vi "alphanumkey_pw.vi"(8 "error in (no error)":errorcluster, 11 "Old Input":string) -> (0 "error out":errorcluster, 3 "Output String":string)   [LabVIEW 2014]
doc: "This VI serves as an on screen keyboard for touch panel modules."
panel:
  in  "Cancel Button":bool
  in  "OK Button":bool
  in  "Boolean":bool
  in  "*":bool
  in  "Delete":bool
  in  "#":bool
  in  "0":bool
  in  ".":bool
  in  "9":bool
  in  "8":bool
  in  "7":bool
  in  "6":bool
  in  "5":bool
  in  "4":bool
  in  "3":bool
  in  "2":bool
  in  "1":bool
  in  "RShift":bool
  in  "Z":bool
  in  "Y":bool
  in  "X":bool
  in  "W":bool
  in  "V":bool
  in  "U":bool
  in  "T":bool
  in  "S":bool
  in  "R":bool
  in  "Q":bool
  in  "P":bool
  in  "O":bool
  in  "N":bool
  in  "M":bool
  in  "L":bool
  in  "K":bool
  in  "J":bool
  in  "I":bool
  in  "H":bool
  in  "G":bool
  in  "F":bool
  in  "E":bool
  in  "D":bool
  in  "C":bool
  in  "B":bool
  in  "LShift":bool
  in  "A":bool
  in  "Blank Button":bool
  in  "stop":bool
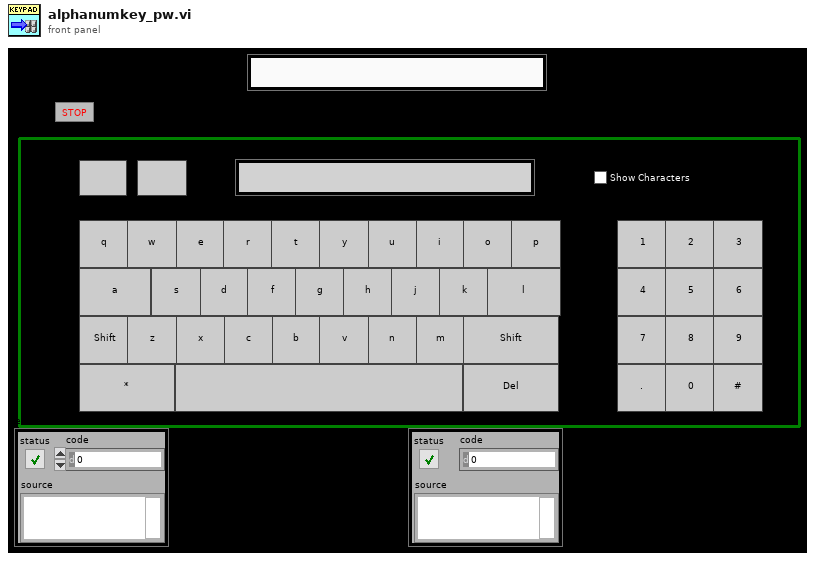
[diagram p1: front panel]
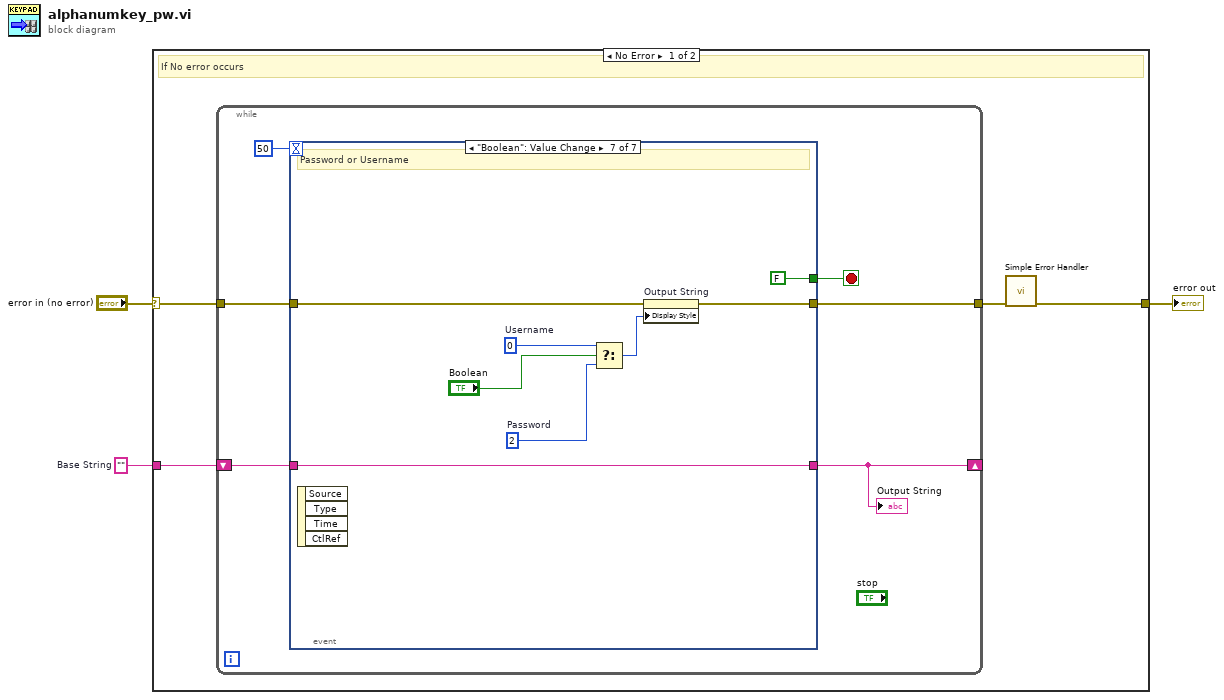
[diagram p0: block diagram]
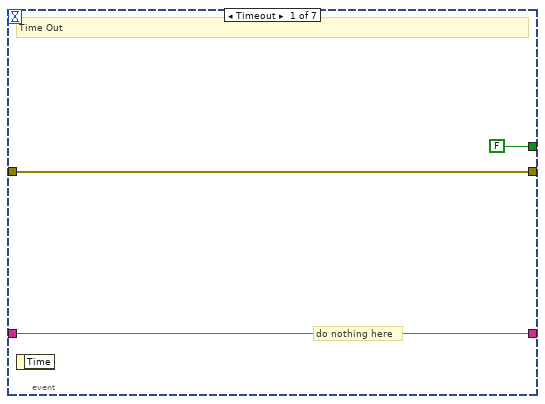
[diagram p2: hidden frame]
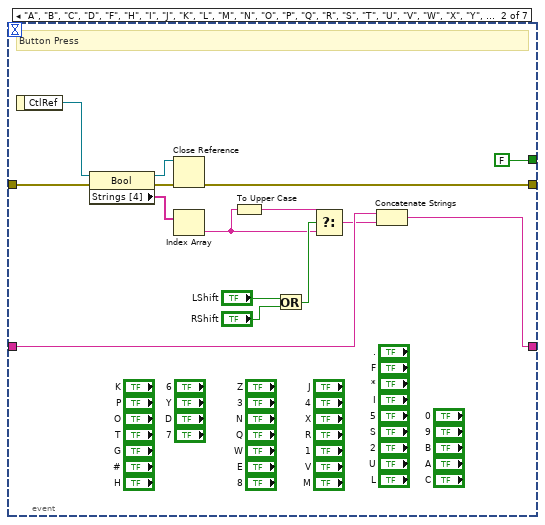
[diagram p3: hidden frame]
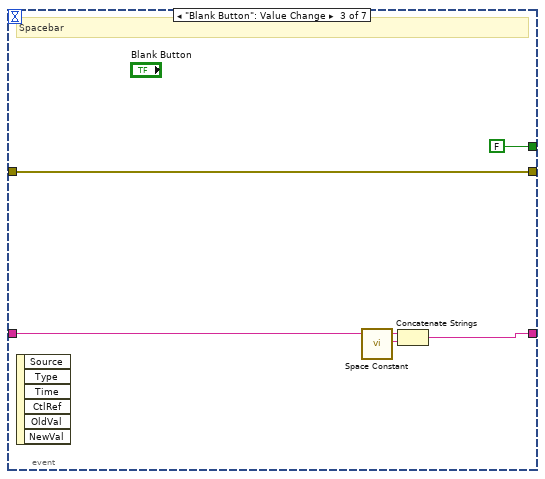
[diagram p4: hidden frame]
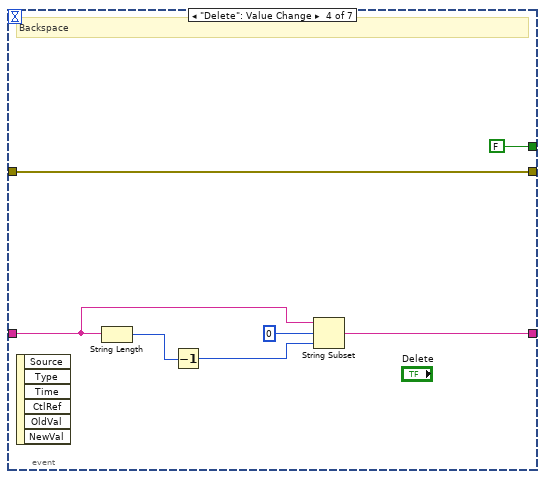
[diagram p5: hidden frame]
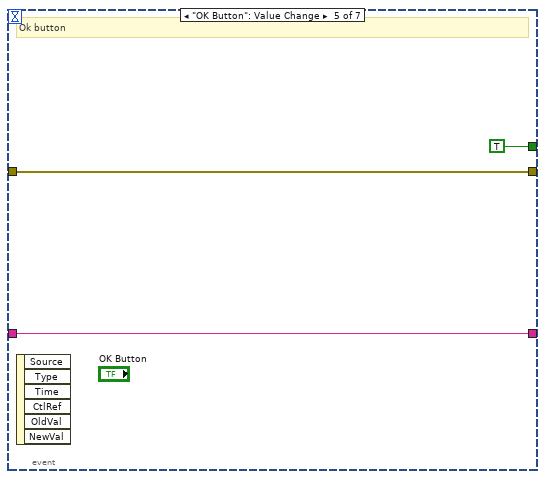
[diagram p6: hidden frame]
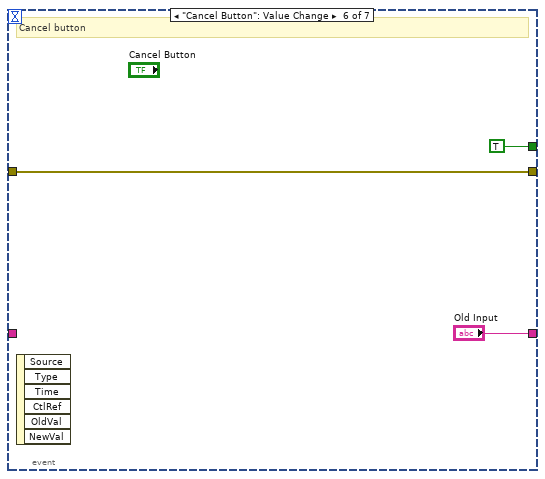
[diagram p7: hidden frame]
diagram:
  w3 = ""  # Base String
  n1 = case shown="No Error" "error in (no error)" {
    selector: "error in (no error)" -> [w4 w58]
    tunnel: w3 -> [w7 _]
    tunnel: [w5 w58] -> w2
    frame No Error {
      # "If No error occurs"
      n2 = while {
        shift-right: [w12] -> _
        shift-left: w7 -> [w11]
        tunnel: [w9] -> w6
        tunnel: w4 -> [w8]
        stop <- w10 stop-if-true
        n3 = event shown="[6] \"Boolean\": Value Change" {
          selector: _ -> [_ _ _ _ _ _ _]
          dyn-events: _ -> [_ _ _ _ _ _ _]
          timeout: 50 -> [_ _ _ _ _ _ _]
          tunnel: [w16 w26 w34 w39 w46 "Old Input" w54] -> w12
          tunnel: w11 -> [w16 w27 w36 w43 w46 _ w54]
          tunnel: [FALSE FALSE FALSE FALSE TRUE TRUE FALSE] -> w10
          tunnel: [w14 w17 w32 w37 w44 w47 w52] -> w9
          tunnel: w8 -> [w14 w18 w32 w37 w44 w47 w51]
          event Timeout {
            # "do nothing here"
            # "Time Out"
            n4 = event-data() -> ()  [unwired: 1 in, 1 out]
          }
          event "A", "B", "C", "D", "F", "H", "I", "J", "K", "L", "M", "N", "O", "P", "Q", "R", "S", "T", "U", "V", "W", "X", "Y", "Z", "1", "2", "3", "4", "5", "6", "7", "8", "9", ".", "0", "#", "E", "G", "*": Value Change {
            # "Button Press"
            n5 = event-data() -> ("CtlRef"=w31:refnum<vi>)  [unwired: 1 in]
            n6 = property class="Bool"(reference=w31, error in=w18) -> (reference out=w29:refnum<vi>, error out=w28:errorcluster, "Strings [4]"=w30:string[])
            n7 = Close Reference(reference=w29, error in (no error)=w28) -> (error out=w17:errorcluster)
            n8 = Index Array(array=w30) -> (element=w20:string)  [unwired: 1 in]
            n9 = To Upper Case(1:w20) -> (0:w25:string)
            n10 = Or(x="LShift", y="RShift") -> (x .or. y?=w21:bool)
            n11 = Select(t=w25, s=w21, f=w20) -> (s? t:f=w24:string)
            n12 = Concatenate Strings(w27, w24) -> (w26:string)
          }
          event "Blank Button": Value Change {
            # "Spacebar"
            n13 = event-data() -> ()  [unwired: 1 in, 6 out]
            n14 = call <vilib>:"Space Constant.vi"() -> ("String"=w35:string)
            n15 = Concatenate Strings(w36, w35) -> (w34:string)
          }
          event "Delete": Value Change {
            # "Backspace"
            n16 = event-data() -> ()  [unwired: 1 in, 6 out]
            n17 = String Length(string=w43) -> (length=w41:i32)
            n18 = Decrement(x=w41) -> (x-1=w40:i32)
            n19 = String Subset(string=w43, offset (0)=0, length (rest)=w40) -> (substring=w39:string)
          }
          event "OK Button": Value Change {
            # "Ok button"
            n20 = event-data() -> ()  [unwired: 1 in, 6 out]
          }
          event "Cancel Button": Value Change {
            # "Cancel button"
            n21 = event-data() -> ()  [unwired: 1 in, 6 out]
          }
          event "Boolean": Value Change {
            w56 = u32 2  # Password
            w57 = u32 0  # Username
            # "Password or Username"
            n22 = event-data() -> ()  [unwired: 1 in, 4 out]
            n23 = Select(t=w57, s="Boolean", f=w56) -> (s? t:f=w55:u32)
            n24 = property on="Output String" class="Str"(error in=w51, "Display Style"=w55) -> (error out=w52:errorcluster)  [unwired: 1 in, 1 out]
          }
        }
        "Output String" <- w12
      }
      n25 = call <vilib>:"Simple Error Handler.vi"("error in (no error)"=w6) -> ("error out"=w5:errorcluster)  [unwired: 4 in, 4 out]
    }
    frame Error {
      # "do nothing"
      # "if an error occurs"
    }
  }
  "error out" <- w2
